vi "Create from CSV.vi"(8 "error in (no error)":errorcluster, 11 "CSV Entries":string[](array[string])) -> (0 "error out":errorcluster, 3 "Banking Statement out":refnum<class "Banking Statement.lvclass">)   [LabVIEW 2018, in "Banking Statement.lvclass"]
uses:
  Banking Statement.lvclass
  C:/Users/jtipps/Documents/Filthy-Lucre-Budgetizer/source/support/classes/Statement/Statement.lvclass
  Statement/Statement.lvclass/Statement.ctl
  Banking Record/Banking Record.lvclass
  C:/Users/jtipps/Documents/Filthy-Lucre-Budgetizer/source/support/classes/Transaction/Transaction.lvclass
  Statement/Statement.lvclass
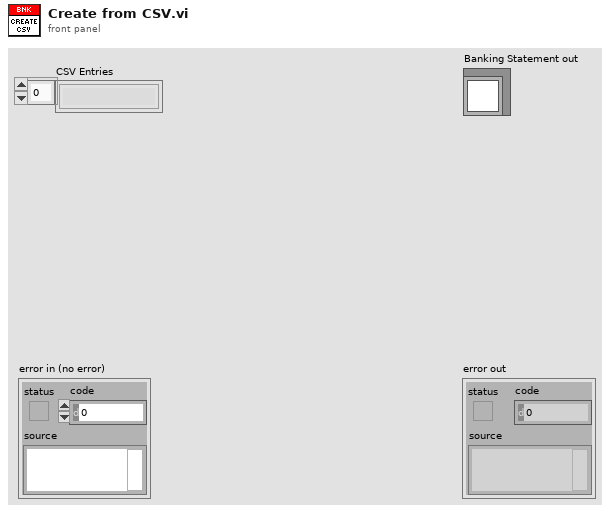
[diagram p1: front panel]
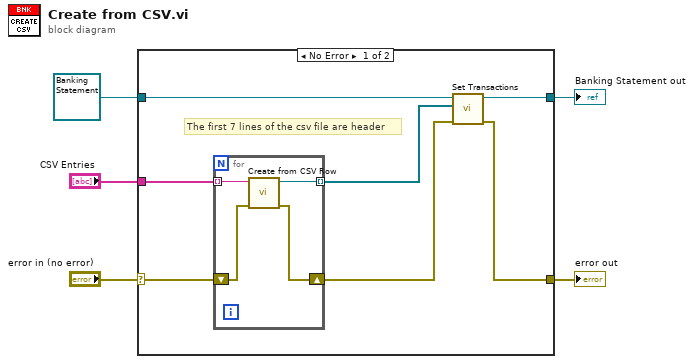
[diagram p0: block diagram]
diagram:
  n1 = case shown="No Error" "error in (no error)" {
    selector: "error in (no error)" -> [w11 w18]
    tunnel: [w7 w18] -> w4
    tunnel: refnum<class "Banking Statement.lvclass"> refnum ("Banking Statement in") -> [w10 w17]
    tunnel: [w9 w17] -> w2
    tunnel: "CSV Entries" -> [w12 _]
    frame No Error {
      # "The first 7 lines of the csv file are header"
      n2 = for {
        tunnel: w12 -> [w15] mode=indexing
        tunnel: [w16] -> w6 mode=indexing
        shift-right: [w13] -> w8
        shift-left: w11 -> [w14]
        n3 = call "Create from CSV Row.vi"("error in (no error)"=w14, "CSV Row"=w15) -> ("error out"=w13:errorcluster, "Banking Record"=w16:refnum<class "Banking Record.lvclass">)  [unwired: 8 in]
      }
      n4 = call "Set Transactions.vi"("error in (no error)"=w8, "Transactions"=w6, "Statement in"=w10) -> ("error out"=w7:errorcluster, "Statement out"=w9:refnum<class "Banking Statement.lvclass">)  [unwired: 7 in]
    }
    frame Error {
    }
  }
  "error out" <- w4
  "Banking Statement out" <- w2
